vi "Update Application Settings.vi"(6 "wait for reply (T)":bool=TRUE, 8 "error in (no error)":errorcluster) -> (0 "error out":errorcluster, 1 "timed out?":bool, 2 "Reply Payload":T1)   [LabVIEW 2018, in "Settings Editor.lvlib"]
doc: "Request Settings Editor to return the latest settings. The Settings Editor can send the applications settings as a reply or via broadcast.\n_____\nCreated using Delacor QMH Event Scripter 4.1.0.75.\n_____\nBased on Delacor QMH Project Template 4.1.0.59."
uses:
  Settings Editor.lvlib
  Update Application Settings (Reply Payload)--cluster.ctl
  Settings--cluster.ctl
  Delacor/PPLs/CML_Shared.lvlibp/Signal Type--enum.ctl
  Delacor/PPLs/CML_Shared.lvlibp/Calibration Values--cluster.ctl
  Update Application Settings Argument--cluster.ctl
  Delacor/PPLs/CML_Shared.lvlibp
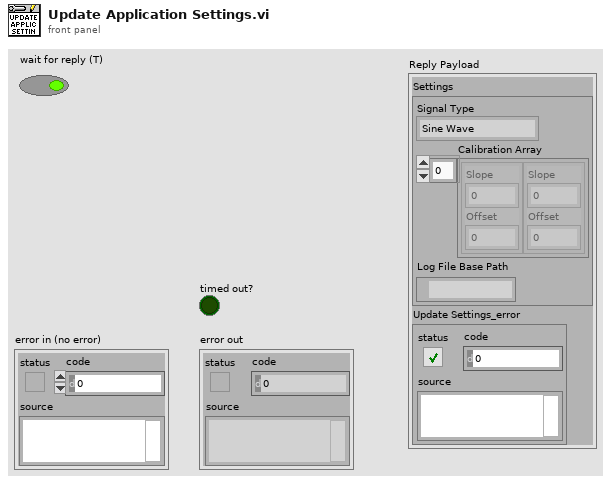
[diagram p1: front panel]
types:
  T1 = typedef "Settings Editor.lvlib/Update Application Settings (Reply Payload)--cluster.ctl" = cluster{"Settings":T2, "Update Settings_error":errorcluster}
  T2 = typedef "Settings Editor.lvlib/Settings--cluster.ctl" = cluster{"Signal Type":T3, "Calibration Array":T4[], "Log File Base Path":path}
  T3 = typedef "CML_Shared.lvlibp/Signal Type--enum.ctl" = enum16{"Sine Wave", "Square with Noise"}
  T4 = typedef "CML_Shared.lvlibp/Calibration Values--cluster.ctl" = cluster{"Slope":dbl, "Offset":dbl}
  T5 = typedef "Settings Editor.lvlib/Request Events--cluster.ctl" = cluster{"Stop Module":refnum<user-event>, "Show Panel":refnum<user-event>, "Hide Panel":refnum<user-event>, "Get Module Execution Status":refnum<user-event>, "Show Diagram":refnum<user-event>, "Update Application Settings":refnum<user-event>}
  T6 = typedef "Settings Editor.lvlib/Update Application Settings Argument--cluster.ctl" = cluster{"Wait Notifier":refnum<notifier>, "wait for reply":bool}
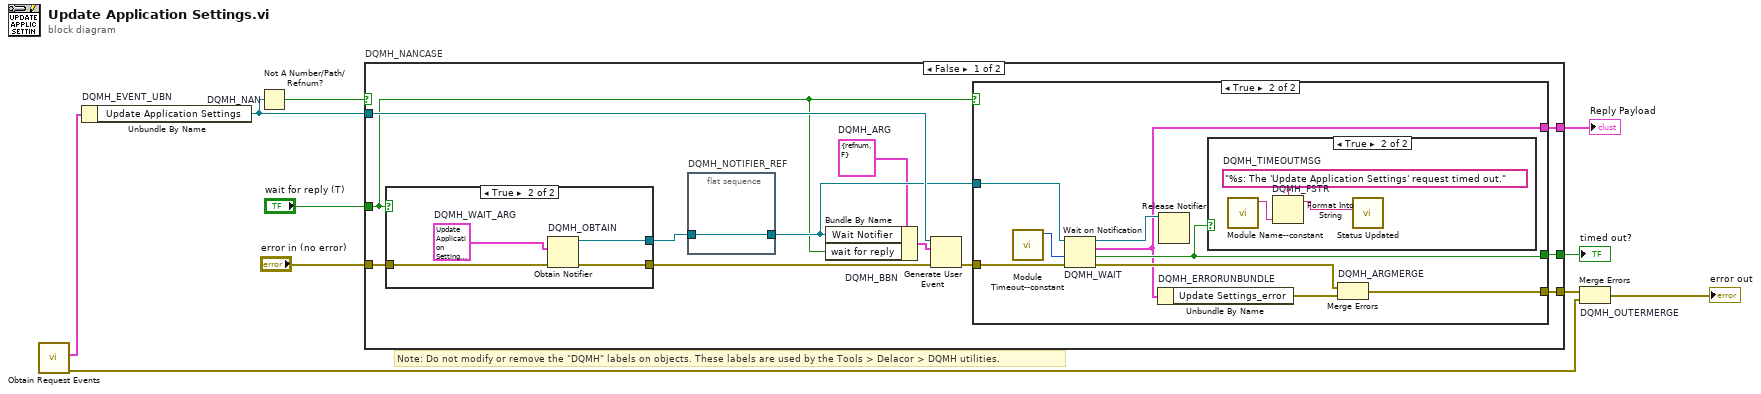
[diagram p0: block diagram]
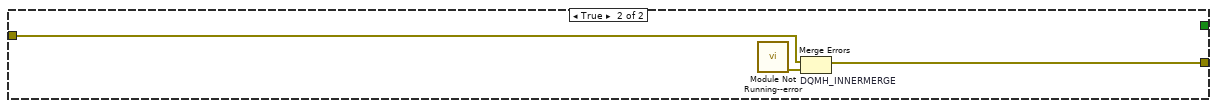
[diagram p5: hidden frame]
diagram:
  # "Note: Do not modify or remove the \"DQMH\" labels on objects. These labels are used by the Tools > Delacor > DQMH utilities."
  n1 = call "Obtain Request Events.vi"() -> ("error out"=w3:errorcluster, "Settings Editor Request Events"=w2:T5)  [unwired: 10 in]
  n2 = Unbundle By Name "DQMH_EVENT_UBN"(w2) -> ("Update Application Settings"=w8:refnum<user-event>)
  n3 = Not A Number/Path/Refnum? "DQMH_NAN"(number/path/refnum=w8) -> (NaN/Path/Refnum?=w7:bool)
  n4 = case "DQMH_NANCASE" shown="False" w7 {
    tunnel: "error in (no error)" -> [w22 w44]
    tunnel: w8 -> [w20 _]
    tunnel: [w17 w43] -> w5
    tunnel: [w18 _] -> w6
    tunnel: "wait for reply (T)" -> [w13 _]
    tunnel: [w11 _] -> w1
    frame False {
      w12 = T6 {"Wait Notifier"=refnum, "wait for reply"=FALSE}  # DQMH_ARG
      n5 = case shown="True" w13 {
        tunnel: w22 -> [w37 w41]
        tunnel: [w37 w40] -> w19
        tunnel: [_ w38] -> w15
        frame False {
        }
        frame True {
          w39 = T1 {"Settings"={"Signal Type"=enum."Sine Wave", "Calibration Array"=[], "Log File Base Path"=path ""}, "Update Settings_error"={"status"=FALSE, "code"=0, "source"=""}}  # DQMH_WAIT_ARG
          n6 = Obtain Notifier "DQMH_OBTAIN"(notification data type=w39, error in (no error)=w41) -> (notifier out=w38:refnum<notifier>, error out=w40:errorcluster)  [unwired: 2 in, 1 out]
        }
      }
      n7 = flat-sequence "DQMH_NOTIFIER_REF" {
        tunnel: w15 -> [w23]
        tunnel: [w23] -> w14
        frame #0 {
        }
      }
      n8 = Bundle By Name "DQMH_BBN"(cluster=w12, "Wait Notifier"=w14, "wait for reply"=w13) -> (w16:T6)
      n9 = Generate User Event(user event=w20, event data cluster=w16, error in=w19) -> (error out=w21:errorcluster)  [unwired: 1 in, 1 out]
      n10 = case shown="True" w13 {
        tunnel: w21 -> [w24 w33]
        tunnel: w14 -> [_ w31]
        tunnel: [_ w29] -> w18
        tunnel: [w24 w28] -> w17
        tunnel: [_ w25] -> w11
        frame False {
        }
        frame True {
          n11 = call "Module Timeout--constant.vi"() -> ("Module Timeout"=w26:i32)  [unwired: 11 in]
          n12 = Wait on Notification "DQMH_WAIT"(notifier=w31, timeout in ms (-1)=w26, error in (no error)=w33) -> (notifier out=w30:refnum<notifier>, notification=w25:T1, timed out?=w29:bool, error out=w32:errorcluster)  [unwired: 1 in]
          n13 = Unbundle By Name "DQMH_ERRORUNBUNDLE"(w25) -> ("Update Settings_error"=w27:errorcluster)
          n14 = Release Notifier(notifier=w30) -> ()  [unwired: 2 in, 3 out]
          n15 = case shown="True" w29 {
            frame False {
            }
            frame True {
              w36 = "%s: The 'Update Application Settings' request timed out."  # DQMH_TIMEOUTMSG
              n16 = call "Module Name--constant.vi"() -> ("Module Name"=w35:string)  [unwired: 11 in]
              n17 = Format Into String "DQMH_FSTR"(format string=w36, w35) -> (resulting string=w34:string)  [unwired: 2 in, 1 out]
              n18 = call "Status Updated.vi"("Status"=w34) -> ()  [unwired: 10 in, 1 out]
            }
          }
          n19 = Merge Errors "DQMH_ARGMERGE"(w32, w27) -> (w28:errorcluster)
        }
      }
    }
    frame True {
      n20 = call "Module Not Running--error.vi"() -> ("error out"=w42:errorcluster)  [unwired: 11 in]
      n21 = Merge Errors "DQMH_INNERMERGE"(w44, w42) -> (w43:errorcluster)
    }
  }
  "timed out?" <- w6
  "Reply Payload" <- w1
  n22 = Merge Errors "DQMH_OUTERMERGE"(w5, w3) -> (→"error out":errorcluster)
